vi "OCR Drone.vi"() -> ()   [LabVIEW 2014]
uses:
  Global.vi
  <vilib>/vision/NI_Vision_Development_Module.lvlib
panel:
  out "Command string":string
  out "State":string
  in  "Reset Button":bool
  out "Land/TakeOff":bool
  out "Get Video Stream Error":errorcluster
  out "OCR":T1(plugin-control)
  out "Number of Lines":i32
  out "Read String":string
  in  "error in (no error)":errorcluster
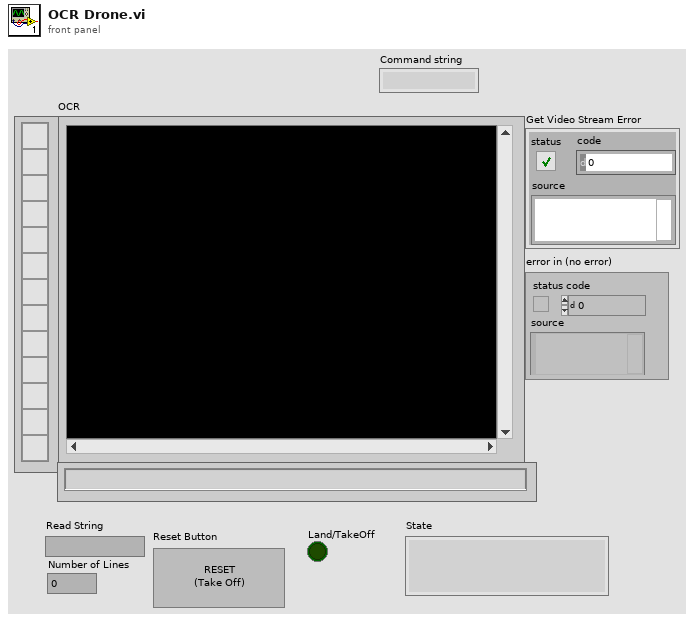
[diagram p1: front panel]
types:
  T1 = typedef "IMAQ Image.ctl" = refnum<image>
  T2 = typedef "Image Type" = u32
  T3 = typedef "IMAQ OCR Session.ctl" = refnum<k1>
  T4 = typedef "Control cluster.ctl" = cluster{"Roll":sgl, "Pitch":sgl, "Vertical Speed":sgl, "Yaw Speed":sgl}
  T5 = cluster{"Global Rectangle":i32[], "Contours":cluster{"ID":enum32{"External", "Internal"}, "Type":u32, "Coordinates":i32[]}[]}
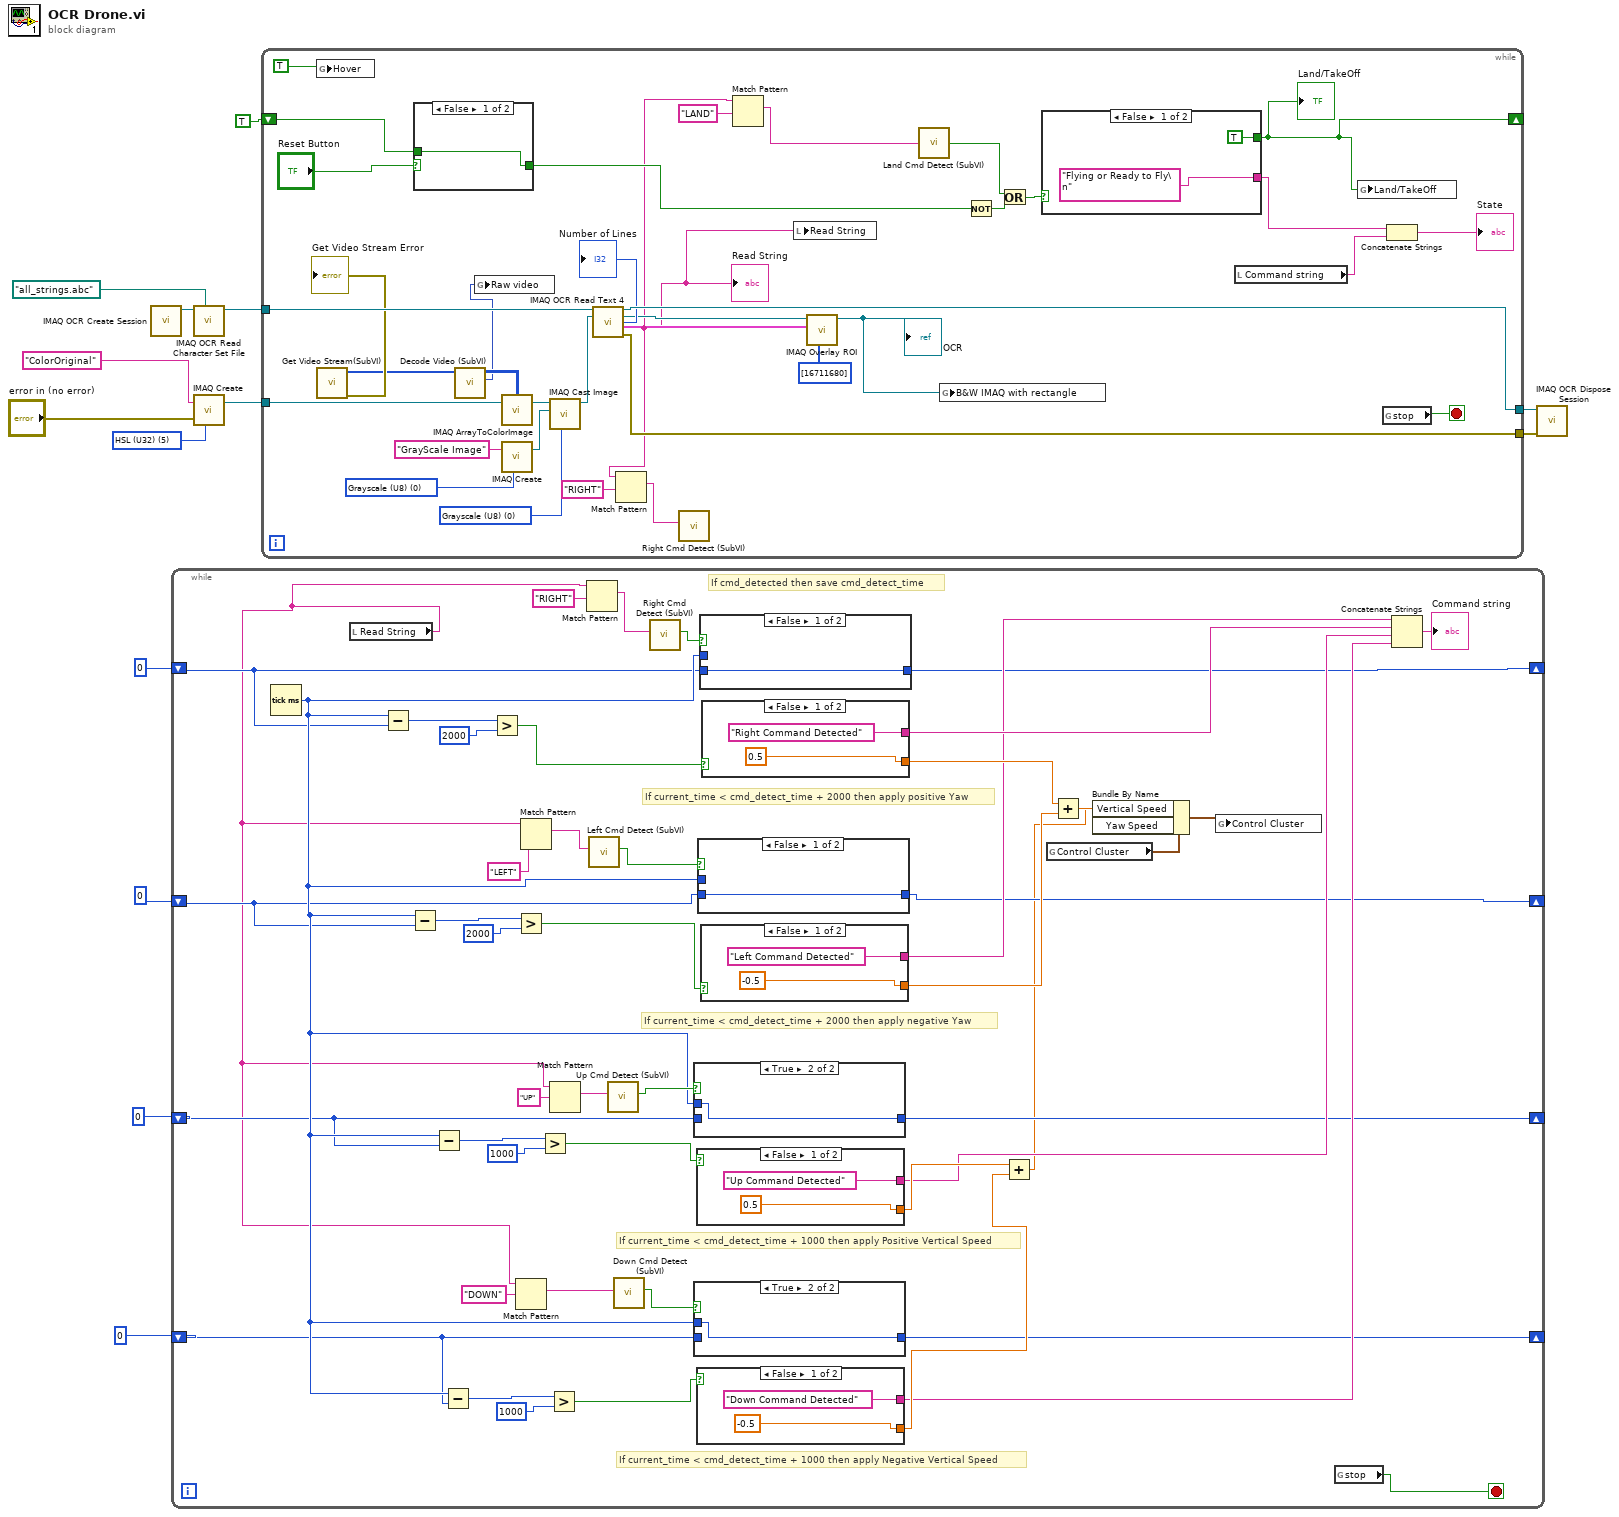
[diagram p0: block diagram]
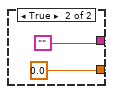
[diagram p2: hidden frame]
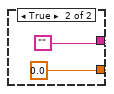
[diagram p4: hidden frame]
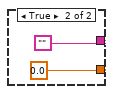
[diagram p6: hidden frame]
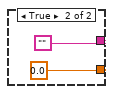
[diagram p8: hidden frame]
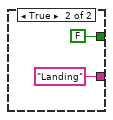
[diagram p11: hidden frame]
diagram:
  w14 = T2 5 items=["Grayscale (U8)", "Grayscale (I16)", "Grayscale (SGL)", "Complex (CSG)", "RGB (U32)", "HSL (U32)", "RGB (U64)", "Grayscale (U16)"] ("Image Type")
  n1 = call "IMAQ OCR Create Session"() -> ("IMAQ OCR Session"=w9:T3)  [unwired: 10 in, 1 out]
  n2 = while {
    shift-right: [w26] -> _
    shift-left: u32 0 ("millisecond timer value") -> [w25]
    shift-right: [w22] -> _
    shift-left: u32 0 ("millisecond timer value") -> [w23]
    shift-right: [w21] -> _
    shift-left: u32 0 ("millisecond timer value") -> [w24]
    shift-right: [w20] -> _
    shift-left: u32 0 ("millisecond timer value") -> [w19]
    stop <- w18 stop-if-true
    # "If current_time < cmd_detect_time + 1000 then apply Negative Vertical Speed"
    # "If current_time < cmd_detect_time + 1000 then apply Positive Vertical Speed"
    # "If current_time < cmd_detect_time + 2000 then apply negative Yaw"
    # "If cmd_detected then save cmd_detect_time"
    # "If current_time < cmd_detect_time + 2000 then apply positive Yaw"
    n3 = Tick Count (ms)() -> (millisecond timer value=w35:u32)
    n4 = local read "Read String"() -> (w17:string)
    n5 = Subtract(x=w35, y=w19) -> (x-y=w60:u32)
    n6 = Subtract(x=w35, y=w23) -> (x-y=w52:u32)
    n7 = Subtract(x=w35, y=w24) -> (x-y=w44:u32)
    n8 = Subtract(x=w35, y=w25) -> (x-y=w36:u32)
    n9 = Greater?(x=w60, y=u32 2000) -> (0:w61:bool)
    n10 = Greater?(x=w52, y=u32 2000) -> (0:w51:bool)
    n11 = Match Pattern(string=w17, regular expression="DOWN") -> (match substring=w32:string)  [unwired: 1 in, 3 out]
    n12 = Match Pattern(string=w17, regular expression="LEFT") -> (match substring=w55:string)  [unwired: 1 in, 3 out]
    n13 = Greater?(x=w44, y=u32 1000) -> (0:w43:bool)
    n14 = Greater?(x=w36, y=u32 1000) -> (0:w34:bool)
    n15 = Match Pattern(string=w17, regular expression="UP") -> (match substring=w42:string)  [unwired: 1 in, 3 out]
    n16 = Match Pattern(string=w17, regular expression="RIGHT") -> (match substring=w46:string)  [unwired: 1 in, 3 out]
    n17 = call "Left Cmd Detect (SubVI).vi"("Read String"=w55) -> ("Left Command"=w54:bool)  [unwired: 10 in]
    n18 = call "Up Cmd Detect (SubVI).vi"("Read String"=w42) -> ("Up Command"=w41:bool)  [unwired: 10 in]
    n19 = call "Down Cmd Detect (SubVI).vi"("Read String"=w32) -> ("Down Command"=w33:bool)  [unwired: 10 in]
    n20 = call "Right Cmd Detect (SubVI).vi"("Read String"=w46) -> ("Right Command"=w47:bool)  [unwired: 10 in]
    n21 = case shown="True" w41 {
      tunnel: [w73 w74] -> w21
      tunnel: w24 -> [w73 _]
      tunnel: w35 -> [_ w74]
      frame False {
      }
      frame True {
      }
    }
    n22 = case shown="True" w33 {
      tunnel: [w67 w68] -> w26
      tunnel: w25 -> [w67 _]
      tunnel: w35 -> [_ w68]
      frame False {
      }
      frame True {
      }
    }
    n23 = case shown="False" w43 {
      tunnel: ["Up Command Detected" ""] -> w29
      tunnel: [0.5 0.0] -> w40
      frame False {
      }
      frame True {
      }
    }
    n24 = case shown="False" w34 {
      tunnel: ["Down Command Detected" ""] -> w30
      tunnel: [-0.5 0.0] -> w38
      frame False {
      }
      frame True {
      }
    }
    n25 = case shown="False" w54 {
      tunnel: [w79 w80] -> w22
      tunnel: w23 -> [w79 _]
      tunnel: w35 -> [_ w80]
      frame False {
      }
      frame True {
      }
    }
    n26 = case shown="False" w47 {
      tunnel: [w85 w86] -> w20
      tunnel: w19 -> [w85 _]
      tunnel: w35 -> [_ w86]
      frame False {
      }
      frame True {
      }
    }
    n27 = case shown="False" w51 {
      tunnel: ["Left Command Detected" ""] -> w27
      tunnel: [-0.5 0.0] -> w49
      frame False {
      }
      frame True {
      }
    }
    n28 = case shown="False" w61 {
      tunnel: ["Right Command Detected" ""] -> w28
      tunnel: [0.5 0.0] -> w50
      frame False {
      }
      frame True {
      }
    }
    n29 = Add(x=w40, y=w38) -> (x+y=w15:dbl)
    n30 = global read "Global.vi" "Control Cluster"() -> (w59:T4)
    n31 = Add(x=w50, y=w49) -> (x+y=w48:dbl)
    n32 = Bundle By Name(cluster=w59, "Vertical Speed"=w15, "Yaw Speed"=w48) -> (w58:T4)
    n33 = global write "Global.vi" "Control Cluster"(w58) -> ()
    n34 = global read "Global.vi" "stop"() -> (w18:bool)
    n35 = Concatenate Strings(w27, w28, w29, w30) -> (→"Command string":string)
  }
  n36 = call "IMAQ OCR Read Character Set File"("File Path"=path "all_strings.abc", "IMAQ OCR Session"=w9) -> ("IMAQ OCR Session (dup)"=w8:T3)  [unwired: 7 in, 2 out]
  n37 = call "IMAQ Create"("Image Name"="ColorOriginal", "Image Type"=w14, "error in (no error)"="error in (no error)") -> ("New Image"=w13:T1)  [unwired: 2 in, 1 out]
  n38 = while {
    tunnel: w13 -> [w109]
    tunnel: [w119] -> w11
    tunnel: [w118] -> w10
    tunnel: w8 -> [w117]
    shift-right: [w101] -> _
    shift-left: TRUE -> [w104]
    stop <- w95 stop-if-true
    w120 = T2 0 items=["Grayscale (U8)", "Grayscale (I16)", "Grayscale (SGL)", "Complex (CSG)", "RGB (U32)", "HSL (U32)", "RGB (U64)", "Grayscale (U16)"] ("Image Type")
    w122 = T2 0 items=["Grayscale (U8)", "Grayscale (I16)", "Grayscale (SGL)", "Complex (CSG)", "RGB (U32)", "HSL (U32)", "RGB (U64)", "Grayscale (U16)"] ("Image Type")
    n39 = global write "Global.vi" "Hover"(TRUE ("Hover")) -> ()
    n40 = call "Get Video Stream(SubVI).vi"() -> ("error out"=→"Get Video Stream Error":errorcluster, "ImgData"=w89:u8[])  [unwired: 10 in]
    n41 = case shown="False" "Reset Button" {
      selector: "Reset Button" -> [_ w124]
      tunnel: w104 -> [w123 _]
      tunnel: [w123 w124] -> w103
      frame False {
      }
      frame True {
      }
    }
    n42 = call "Decode Video (SubVI).vi"("ImgData"=w89) -> ("new picture"=w87:picture, "Array"=w88:u32[][])  [unwired: 9 in]
    n43 = global write "Global.vi" "Raw video"(w87) -> ()
    n44 = call "IMAQ ArrayToColorImage"("Image Pixels (U32)"=w88, "Image"=w109) -> ("Image Out"=w110:T1)  [unwired: 3 in, 1 out]
    n45 = call "IMAQ Create"("Image Name"="GrayScale Image", "Image Type"=w120) -> ("New Image"=w113:T1)  [unwired: 3 in, 1 out]
    n46 = call "IMAQ Cast Image"("Image Type"=w122, "Image Dst"=w113, "Image Src"=w110) -> ("Image Dst Out"=w112:T1)  [unwired: 7 in, 1 out]
    n47 = call "IMAQ OCR Read Text 4"("IMAQ OCR Session"=w117, "Image"=w112) -> ("IMAQ OCR Session (dup)"=w118:T3, "Image (dup)"=w111:T1, "Number of Lines"=→"Number of Lines":i32, "Read String"=w93:string, "ROI Bounding Characters"=w115:T5, "error out"=w119:errorcluster)  [unwired: 7 in, 1 out]
    "Read String" <- w93
    n48 = Match Pattern(string=w93, regular expression="RIGHT") -> (match substring=w96:string)  [unwired: 1 in, 3 out]
    n49 = call "Right Cmd Detect (SubVI).vi"("Read String"=w96) -> ()  [unwired: 10 in, 1 out]
    n50 = Match Pattern(string=w93, regular expression="LAND") -> (match substring=w97:string)  [unwired: 1 in, 3 out]
    n51 = local write "Read String"(w93) -> ()
    n52 = call "IMAQ Overlay ROI"("Colors (Green)"=u32[] [16711680], "ROI Descriptor"=w115, "Image"=w111) -> ("Image Out"=w94:T1)  [unwired: 7 in, 1 out]
    "OCR" <- w94
    n53 = call "Land Cmd Detect (SubVI).vi"("Read String"=w97) -> ("Land Command"=w102:bool)
    n54 = global write "Global.vi" "B&W IMAQ with rectangle"(w94) -> ()
    n55 = Not(x=w103) -> (.not. x?=w106:bool)
    n56 = Or(x=w102, y=w106) -> (x .or. y?=w107:bool)
    n57 = case shown="False" w107 {
      tunnel: [TRUE FALSE] -> w101
      tunnel: ["Flying or Ready to Fly\n" "Landing"] -> w92
      frame False {
      }
      frame True {
      }
    }
    "Land/TakeOff" <- w101
    n58 = local read "Command string"() -> (w90:string)
    n59 = global write "Global.vi" "Land/TakeOff"(w101) -> ()
    n60 = global read "Global.vi" "stop"() -> (w95:bool)
    n61 = Concatenate Strings(w92, w90) -> (→"State":string)
  }
  n62 = call "IMAQ OCR Dispose Session"("error in (no error)"=w11, "IMAQ OCR Session"=w10) -> ()  [unwired: 9 in, 1 out]
